vi "Get BufferLossless.vi"(11 "AI Voltage DAQmx Cont CFG in":refnum<class "AI Voltage DAQmx Cont CFG.lvclass">) -> (2 "BufferLossless":refnum<class "BufferLossless.lvclass">, 3 "AI Voltage DAQmx Cont CFG out":refnum<class "AI Voltage DAQmx Cont CFG.lvclass">)   [LabVIEW 2024, in "AI Voltage DAQmx Cont CFG.lvclass"]
uses:
  AI Voltage DAQmx Cont CFG.lvclass
  Buffers/BufferLossless/BufferLossless.lvclass
  AI Voltage DAQmx Cont CFG.lvclass/AI Voltage DAQmx Cont CFG.ctl
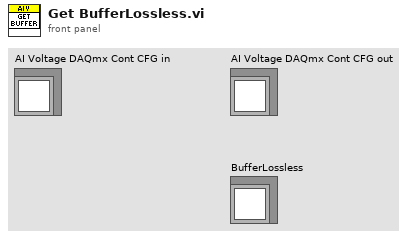
[diagram p1: front panel]
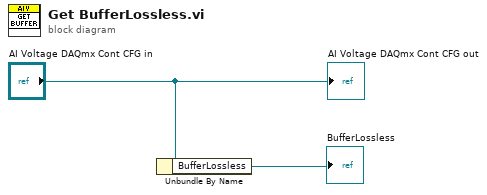
[diagram p0: block diagram]
diagram:
  n1 = Unbundle By Name("AI Voltage DAQmx Cont CFG in") -> ("BufferLossless"=→"BufferLossless":refnum<class "BufferLossless.lvclass">)
  "AI Voltage DAQmx Cont CFG out" <- "AI Voltage DAQmx Cont CFG in"
